vi "util_get_array_element.vi"(5 "Value unit":string="V", 7 "Value name":string="correction for voltage", 8 "error in (no error)":errorcluster, 10 "Desired element":dbl=2.5 format="%#_13g", 11 "Array":dbl[](array[numeric])) -> (0 "error out":errorcluster, 2 "New index":i32)   [LabVIEW 2016]
doc: "Search array for value and return index of first occurance if found. If not, propose the two closest values instead in a dialog. Defaults to skip after timeout."
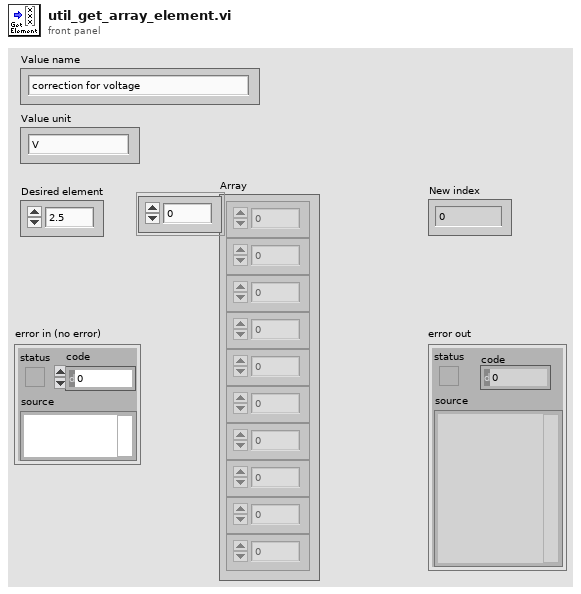
[diagram p1: front panel]
types:
  T1 = enum16{"Left Button", "Center Button", "Right Button", "Window Close"}
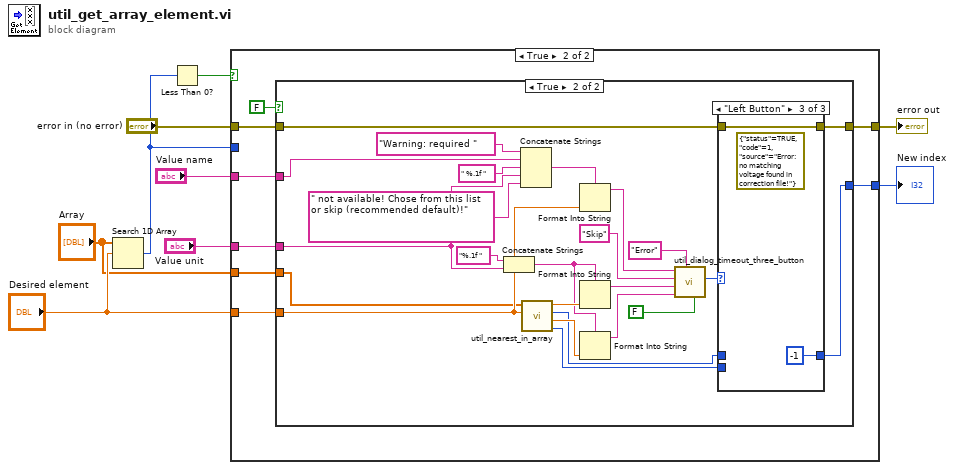
[diagram p0: block diagram]
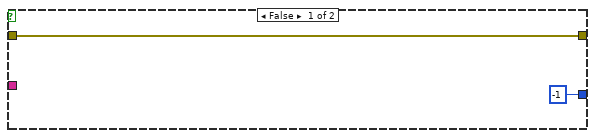
[diagram p3: hidden frame]
diagram:
  n1 = Search 1D Array(1D array="Array", element="Desired element") -> (index of element=w7:i32)  [unwired: 1 in]
  n2 = Less Than 0?(x=w7) -> (x < 0?=w9:bool)
  n3 = case shown="True" w9 {
    tunnel: w7 -> [w11 _]
    tunnel: [w11 w17] -> w8
    tunnel: "Array" -> [_ w18]
    tunnel: "Desired element" -> [_ w19]
    tunnel: "error in (no error)" -> [w10 w16]
    tunnel: [w10 w15] -> w3
    tunnel: "Value name" -> [_ w13]
    tunnel: "Value unit" -> [_ w12]
    frame False {
    }
    frame True {
      n4 = case shown="True" FALSE {
        tunnel: w19 -> [_ w45]
        tunnel: w18 -> [_ w44]
        tunnel: [-1 ("2nd closest index") w39] -> w17
        tunnel: w16 -> [w21 w38]
        tunnel: [w21 w37] -> w15
        tunnel: w13 -> [_ w28]
        tunnel: w12 -> [_ w22]
        frame False {
        }
        frame True {
          n5 = Concatenate Strings("%.1f " ("format string"), w22) -> (w24:string)
          n6 = Concatenate Strings("Warning: required " ("Window Title (\"\")"), w28, " %.1f " ("string"), w22, " not available! Chose from this list or skip (recommended default)!" ("Window Title (\"\")")) -> (w25:string)
          n7 = call "util_nearest_in_array.vi"("desired element"=w45, "1D Array"=w44) -> ("2nd closest index"=w41:i32, "2nd closest element"=w42:dbl, "closest index"=w40:i32, "closest element"=w43:dbl)  [unwired: 6 in]
          n8 = Format Into String(format string=w25, w45) -> (resulting string=w35:string)  [unwired: 2 in, 1 out]
          n9 = Format Into String(format string=w24, w43) -> (resulting string=w31:string)  [unwired: 2 in, 1 out]
          n10 = Format Into String(format string=w24, w42) -> (resulting string=w32:string)  [unwired: 2 in, 1 out]
          n11 = call "util_dialog_timeout_three_button.vi"("Allow user to close window? (TRUE)"=FALSE, "Window Title (\"\")"="Error" ("Window Title (\"\")"), "Right Button Text (\"Cancel\")"=w32, "Center Button Text (\"No\")"=w31, "Default Button Text (\"Yes\")"="Skip" ("Default Button Text (\"Yes\")"), "message"=w35) -> ("Which Button?"=w33:T1)  [unwired: 5 in]
          n12 = case shown="\"Left Button\"" w33 {
            tunnel: w40 -> [w47 _ _]
            tunnel: w41 -> [_ w49 _]
            tunnel: [w47 w49 -1] -> w39
            tunnel: w38 -> [w46 w48 w50]
            tunnel: [w46 w48 w50] -> w37
            frame "Center Button", Default {
            }
            frame "Right Button" {
            }
            frame "Left Button" {
              (unwired) errorcluster {"status"=TRUE, "code"=1, "source"="Error: no matching voltage found in correction file!"} ("error constant")
            }
          }
        }
      }
    }
  }
  "New index" <- w8
  "error out" <- w3
